vi "Create Channel.vi"(5 "Input terminals configurations":T1[](array[typedef]), 7 "Ranges":T3[](array[typedef]), 8 "error in (no error)":errorcluster, 10 "Phisical channels":T2[](array[typedef]) items=["AI1", "AI2", "AI3", "AI4", "AI5", "AI6", "AI7", "AI8", "AI9", "AI10", "AI11", "AI12", "AI13", "AI14", "AI15", "AI16"], 11 "connection ID":i32=-1) -> (0 "error out":errorcluster, 3 "Task Out":refnum<class "Analog Input.lvclass">)   [LabVIEW 2009, in "MicroDAQ.lvlib" / "Analog Input.lvclass"]
doc: "Creates channel(s) to measure voltage. Use Configure channel.VI to specify Sample Rate, Blocking settings."
uses:
  <instrlib>/MicroDAQ/Channel/Analog Input/Analog Input.lvclass
  <instrlib>/MicroDAQ/Tools/Analo Range Enum.ctl
  <instrlib>/MicroDAQ/Tools/Analog input Channel enum.ctl
  <instrlib>/MicroDAQ/Tools/Analog input type enum.ctl
  <instrlib>/MicroDAQ/Channel/Analog Input/Analog Input.lvclass/Analog Input.ctl
  <instrlib>/MicroDAQ/Channel/Channel.lvclass
  <instrlib>/MicroDAQ/MicroDAQ.lvlib
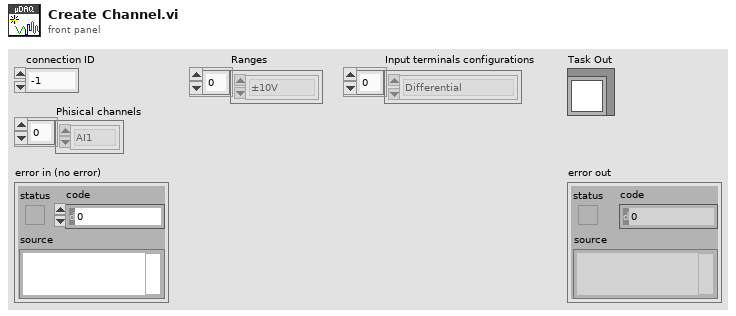
[diagram p1: front panel]
types:
  T1 = typedef "MicroDAQ.lvlib/Analog input type enum.ctl" = enum8{"Single-ended", "Differential"}
  T2 = typedef "MicroDAQ.lvlib/Analog input Channel enum.ctl" = u16
  T3 = typedef "MicroDAQ.lvlib/Analo Range Enum.ctl" = enum16{"±10V", "0-10V", "±5V", "0-5V", "±5.12V", "±2.56V", "±2.5V", "±2V", "±1.24V", "±0.64V"}
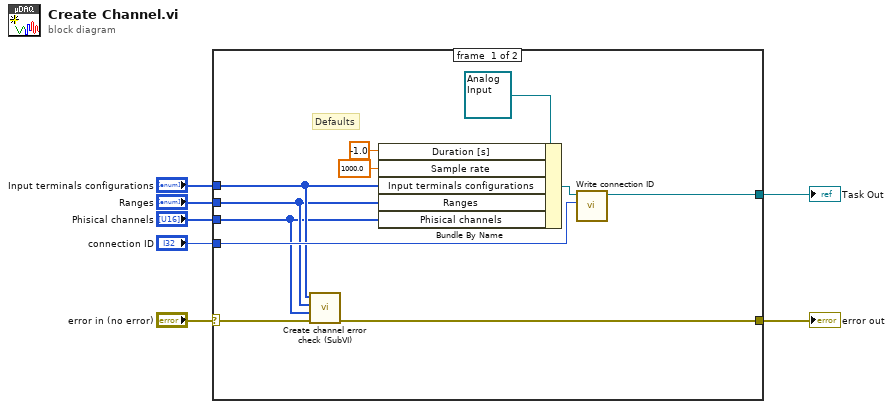
[diagram p0: block diagram]
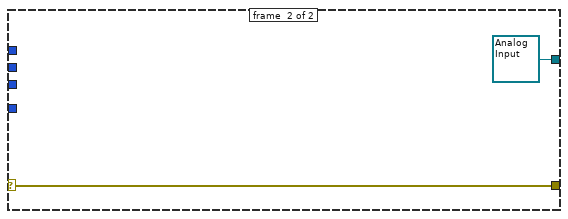
[diagram p2: hidden frame]
diagram:
  n1 = case shown="No Error" "error in (no error)" {
    selector: "error in (no error)" -> [w9 w20]
    tunnel: [w8 w20] -> w6
    tunnel: "Phisical channels" -> [w10 _]
    tunnel: "Ranges" -> [w11 _]
    tunnel: "connection ID" -> [w15 _]
    tunnel: [w14 refnum<class "Analog Input.lvclass"> refnum ("Task out")] -> w2
    tunnel: "Input terminals configurations" -> [w12 _]
    frame #0 {
      # "Defaults"
      n2 = call <instrlib>:"Create channel error check (SubVI).vi"("error in (no error)"=w9, "Phisical channels"=w10, "Ranges"=w11, "Input terminals configurations"=w12) -> ("error out"=w8:errorcluster)  [unwired: 7 in]
      n3 = Bundle By Name(cluster=refnum<class "Analog Input.lvclass"> refnum ("MicroDAQ.lvlib:Analog Input.lvclass"), "Duration [s]"=-1.0 ("duration"), "Sample rate"=1000.0 ("rate"), "Input terminals configurations"=w12, "Ranges"=w11, "Phisical channels"=w10) -> (w18:refnum<class "Analog Input.lvclass">)
      n4 = call <instrlib>:"Write connection ID.vi"("connection ID"=w15, "Task in"=w18) -> ("Task out"=w14:refnum<class "Analog Input.lvclass">)  [unwired: 9 in]
    }
    frame #1 {
    }
  }
  "error out" <- w6
  "Task Out" <- w2
